vi "Read Config File Section.vi"(7 "Section":string, 8 "error in (no error)":errorcluster, 10 "create file if necessary? (F)":bool, 11 "appended path":path) -> (0 "error out":errorcluster, 1 "Values":string[](array[string]), 2 "Keys":string[](array[string]))   [LabVIEW 2018]
uses:
  <vilib>/Utility/config.llb/Read Key (String).vi
  <vilib>/Utility/config.llb/NI_LVConfig.lvlib
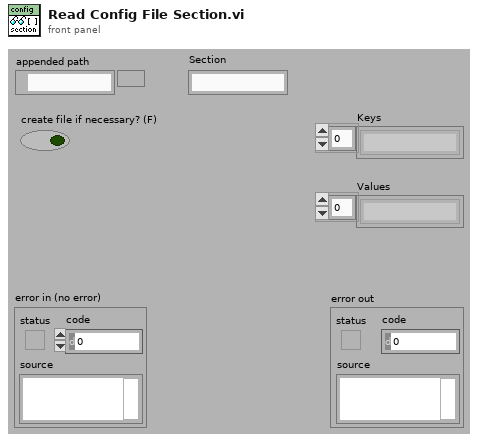
[diagram p1: front panel]
types:
  T1 = typedef "NI_LVConfig.lvlib/Config Data RefNum.ctl" = refnum<k1>
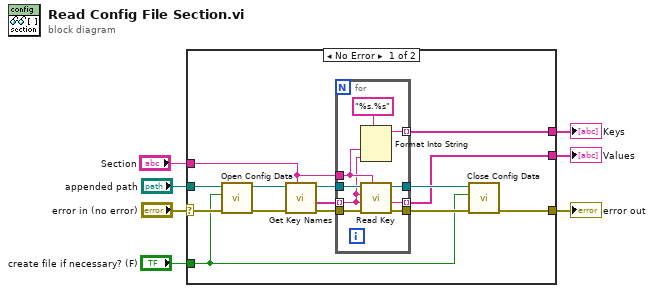
[diagram p0: block diagram]
diagram:
  n1 = case shown="No Error" "error in (no error)" {
    selector: "error in (no error)" -> [w17 w31]
    tunnel: "appended path" -> [w21 _]
    tunnel: [w9 _] -> w6
    tunnel: [w8 _] -> w5
    tunnel: [w20 w31] -> w4
    tunnel: "create file if necessary? (F)" -> [w16 _]
    tunnel: "Section" -> [w10 _]
    frame No Error {
      n2 = call <vilib>:"Open Config Data.vi"("error in (no error)"=w17, "create file if necessary (T)"=w16, "configuration file path"=w21) -> ("error out"=w12:errorcluster, "refnum"=w11:T1)  [unwired: 6 in, 1 out]
      n3 = call <vilib>:"Get Key Names.vi"("section"=w10, "error in (no error)"=w12, "refnum"=w11) -> ("error out"=w14:errorcluster, "key names"=w13:string[], "refnum out"=w15:T1)  [unwired: 5 in, 1 out]
      n4 = for {
        tunnel: w15 -> [w30]
        tunnel: w13 -> [w23] mode=indexing
        tunnel: [w29] -> w8 mode=indexing
        tunnel: [w28] -> w19
        tunnel: w14 -> [w27]
        tunnel: [w26] -> w18
        tunnel: w10 -> [w24]
        tunnel: [w22] -> w9 mode=indexing
        n5 = Format Into String(format string="%s.%s", w24, w23) -> (resulting string=w22:string)  [unwired: 2 in, 1 out]
        n6 = call-poly <vilib>:"Read Key.vi"("section"=w24, "error in (no error)"=w27, "default value"=w23, "key"=w23, "refnum"=w30) -> ("error out"=w26:errorcluster, "value"=w29:string, "refnum out"=w28:T1)  [unwired: 3 in, 1 out]
      }
      n7 = call <vilib>:"Close Config Data.vi"("error in (no error)"=w18, "write file if changed (T)"=w16, "refnum"=w19) -> ("error out"=w20:errorcluster)  [unwired: 7 in, 1 out]
    }
    frame Error {
    }
  }
  "Keys" <- w6
  "Values" <- w5
  "error out" <- w4
